vi "Day 22-Add Intersection.vi"(9 "Sign":i64, 10 "Intersection in":i64[](array[numeric]), 11 "Map in":map{i64[], i64}(c390)) -> (3 "Map out":map{i64[], i64}(c390))   [LabVIEW 2021]
uses:
  <vilib>/Utility/miscctls.llb/LVMapReplaceAction.ctl
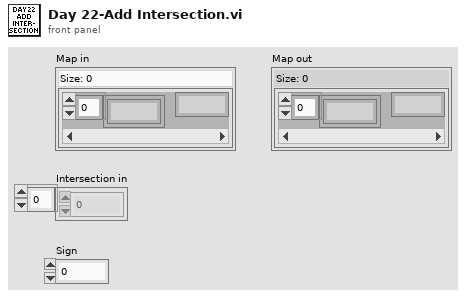
[diagram p1: front panel]
types:
  T1 = typedef "LVMapReplaceAction.ctl" = enum32{"Modify Entry only if found", "Add or Modify Entry", "Delete Entry"}
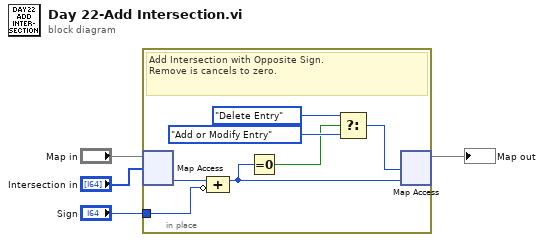
[diagram p0: block diagram]
diagram:
  n1 = in-place {
    in-place-border: "Sign" -> [w5]
    # "Add Intersection with Opposite Sign. \nRemove is cancels to zero."
    n2 = in-place-map #1("Map in", "Intersection in") -> (w11:i64)  [unwired: 1 in, 1 out]
    n3 = Compound Arithmetic op=ADD(w11, invert w5) -> (w10:i64)
    n4 = Equal To 0?(x=w10) -> (x = 0?=w6:bool)
    n5 = Select(t=LVMapReplaceAction."Delete Entry" ("action"), s=w6, f=LVMapReplaceAction."Add or Modify Entry" ("action")) -> (s? t:f=w8:T1)
    n6 = in-place-map #1(w10, w8) -> (→"Map out":map{i64[], i64})  [unwired: 2 out]
  }
